vi "Data Channel Page.vi"(8 "error in (no error)":errorcluster, 11 "Node Ptr":T2 format="%.0x") -> (0 "error out":errorcluster)   [LabVIEW 2019, in "DSF System Explorer.lvlib"]
uses:
  DSF System Explorer.lvlib
  <vilib>/NI VeriStand/Custom Device API/Custom Device API.lvlib
  Shared/DSF Shared.lvlib
  DSF Core.lvlibp/Classes/Component User Interface/UI Type.ctl
  <vilib>/NI VeriStand/Custom Device API/Custom Device Item Ref.ctl
panel:
  in  "Tab Control":enum32{"Settings"}(tab)
  in  "Default Value":dbl
  in  "Units":string
  out "Direction":enum16{"Tx", "Rx"}(ring)
  in  "Engine Data Type":T1(ring)
  in  "String Data Type":T1(ring)
  in  "String Offset":u64 format="%d bytes"
  in  "Header":cluster{"Section Name":string}={"Section Name"="Data Channel"}
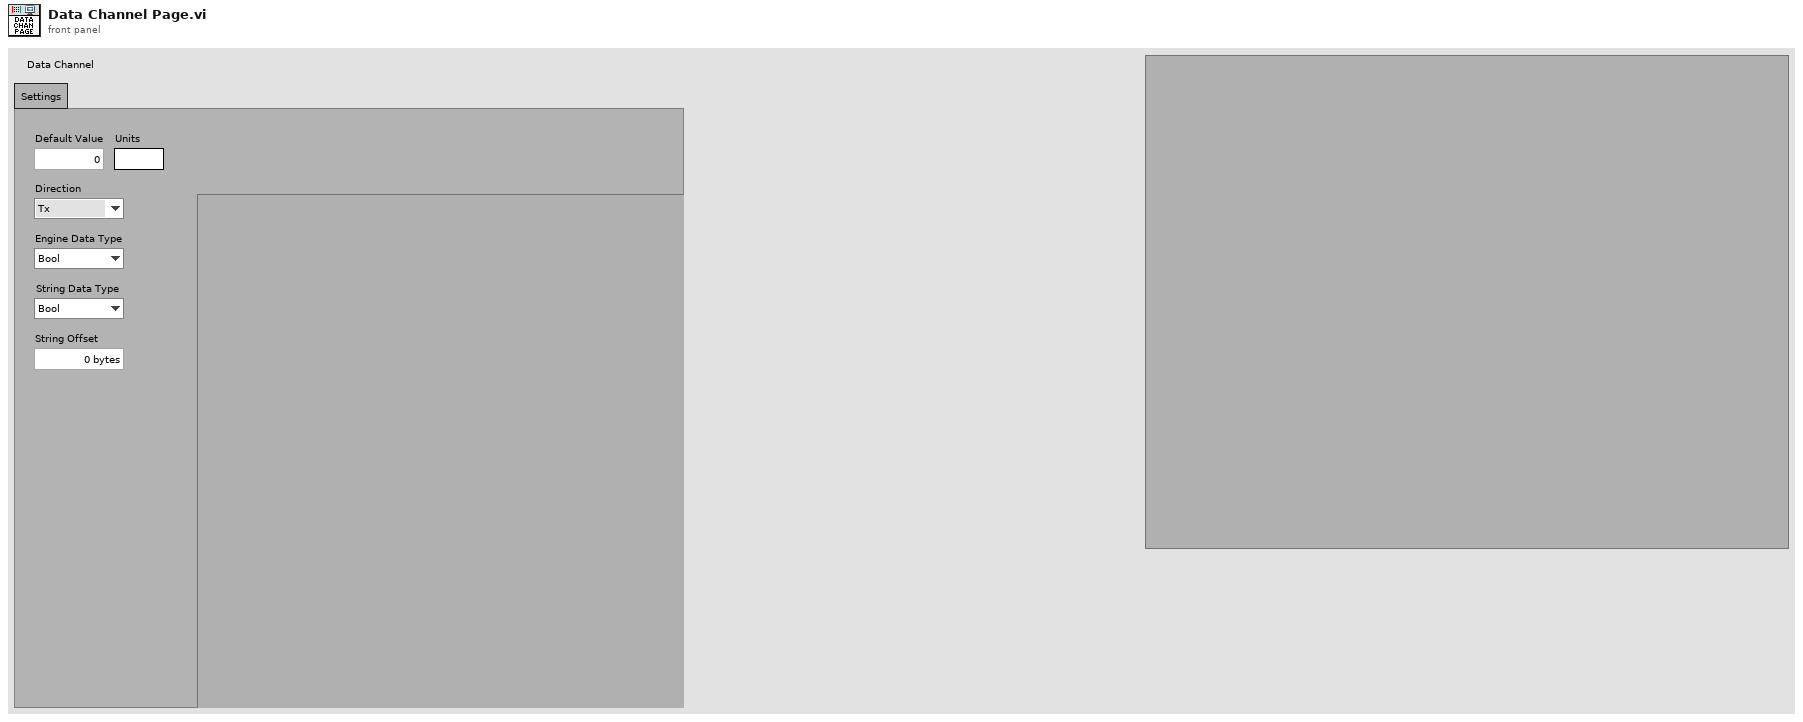
[diagram p1: front panel]
types:
  T1 = enum8{"Bool", "SGL", "DBL", "I8", "I16", "I32", "I64", "U8", "U16", "U32", "U64"}
  T2 = typedef "Custom Device API.lvlib/Custom Device Item Ref.ctl" = u64
  T3 = typedef "DSF Core.lvlibp/Component User Interfaces.lvclass/UI Type.ctl" = enum16{"Plugin", "Thread", "Rx Group", "Tx Group", "Rx Transfer", "Tx Transfer", "Rx Channel", "Tx Channel"}
  T4 = typedef "DSF Core.lvlibp/Channel Configuration.lvclass/Core Channel Configuration.ctl" = cluster{"name":string, "units":string, "engine data type":T5, "string data type":T5, "string offset":u64}
  T5 = typedef "DSF Core.lvlibp/DSF Data Type.ctl" = enum8{"Bool", "SGL", "DBL", "I8", "I16", "I32", "I64", "U8", "U16", "U32", "U64"}
  T6 = typedef "Custom Device API.lvlib/Custom Device Channel.ctl" = cluster{"Type":T7, "Units":string, "Default Value":dbl, "Faultable":bool, "Scalable":bool}
  T7 = typedef "Custom Device API.lvlib/Custom Device Channel Type.ctl" = enum16{"Input", "Output"}
  T8 = typedef "DSF Core.lvlibp/DSF Direction.ctl" = enum8{"Tx", "Rx"}
  T9 = typedef "DSF Core.lvlibp/User Interface Handler.lvclass/User Interface Ref.ctl" = refnum<vi>
  T10 = typedef "DSF Core.lvlibp/DSF Settings Info.ctl" = cluster{"component":string, "values":cluster{"key":string, "value":string}[]}
  T11 = typedef "Custom Device API.lvlib/Custom Device Commands.ctl" = enum16{"Default", "Item renamed", "Shutdown", "Dynamic button pressed"}
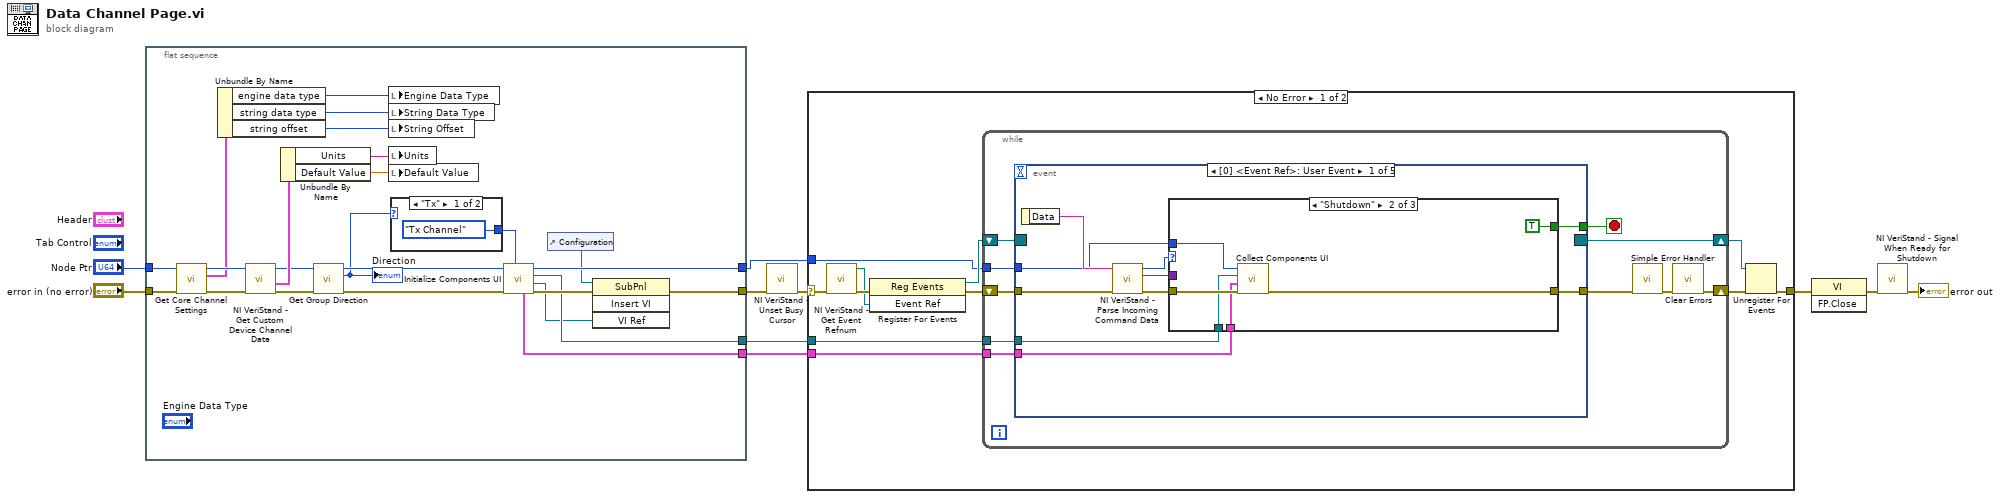
[diagram p0: block diagram]
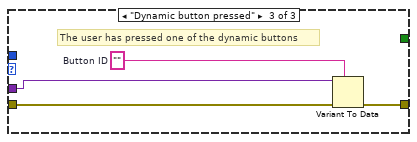
[diagram p3: hidden frame]
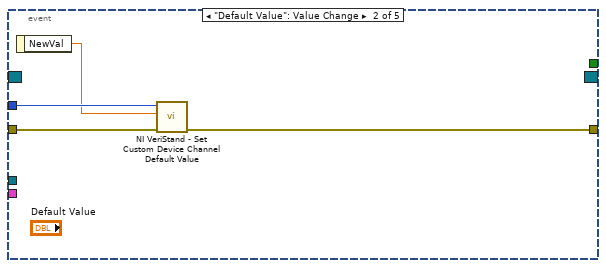
[diagram p4: hidden frame]
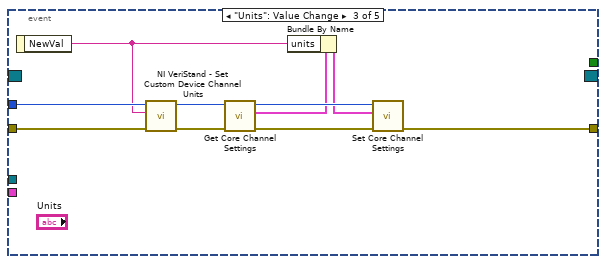
[diagram p5: hidden frame]
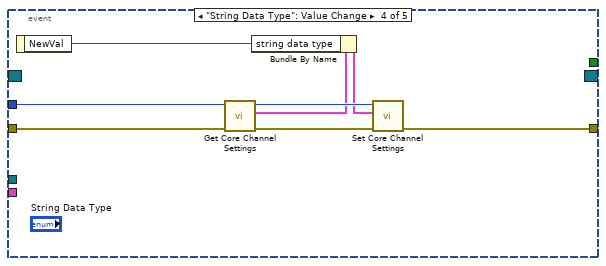
[diagram p6: hidden frame]
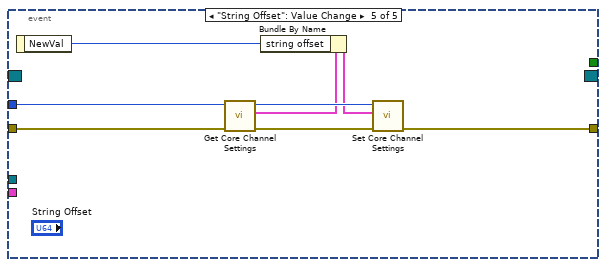
[diagram p7: hidden frame]
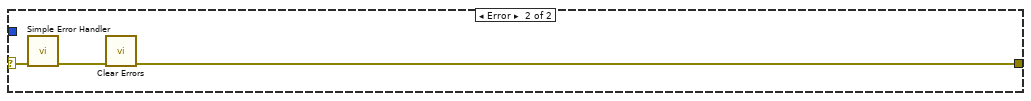
[diagram p8: hidden frame]
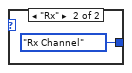
[diagram p9: hidden frame]
diagram:
  n1 = flat-sequence "Initialization code" {
    tunnel: "error in (no error)" -> [w32]
    tunnel: "Node Ptr" -> [w31]
    tunnel: [w19] -> w6
    tunnel: [w14] -> w3
    tunnel: [w15] -> w2
    tunnel: [w11] -> w1
    frame #0 {
      n2 = call "Get Core Channel Settings.vi"("error in (no error)"=w32, "Item Ref in"=w31) -> ("error out"=w30:errorcluster, "channel configuration"=w28:T4, "Item Ref out"=w29:T2)  [unwired: 7 in]
      n3 = Unbundle By Name(w28) -> ("engine data type"=w26:T5, "string data type"=w25:T5, "string offset"=w24:u64)
      n4 = call <vilib>:"NI VeriStand - Get Custom Device Channel Data.vi"("error in (no error)"=w30, "Channel Ref in"=w29) -> ("error out"=w23:errorcluster, "Channel"=w27:T6, "Channel Ref out"=w22:T2)  [unwired: 4 in, 3 out]
      n5 = Unbundle By Name(w27) -> ("Units"=w33:string, "Default Value"=w34:dbl)
      n6 = call "Get Group Direction.vi"("error in (no error)"=w23, "Item Ref in"=w22) -> ("error out"=w18:errorcluster, "direction"=w16:T8, "Item Ref out"=w17:T2)  [unwired: 6 in, 1 out]
      "Direction" <- w16
      n7 = local write "Engine Data Type"(w26) -> ()
      n8 = local write "String Data Type"(w25) -> ()
      n9 = local write "String Offset"(w24) -> ()
      n10 = local write "Units"(w33) -> ()
      n11 = local write "Default Value"(w34) -> ()
      n12 = case shown="\"Tx\"" w16 {
        tunnel: [UI_Type."Tx Channel" ("user interface type") UI_Type."Rx Channel" ("user interface type")] -> w21
        frame "Tx" {
        }
        frame "Rx" {
        }
      }
      n13 = call "Initialize Components UI.vi"("user interface type"=w21, "error in (no error)"=w18, "Item Ref in"=w17) -> ("error out"=w20:errorcluster, "active vi"=w13:T9, "User Interface Handler"=w15:refnum<class "User Interface Handler.lvclass">, "Item Ref out"=w14:T2, "component settings"=w11:T10[])  [unwired: 4 in]
      n14 = control-ref of="Configuration"() -> (w12:refnum<vi>)
      n15 = invoke class="SubPnl" method="Insert VI"(reference=w12, error in=w20, "VI Ref"=w13) -> (error out=w19:errorcluster)  [unwired: 1 in, 3 out]
    }
  }
  n16 = call <vilib>:"NI VeriStand - Unset Busy Cursor.vi"("error in (no error)"=w6) -> ("error out"=w5:errorcluster)  [unwired: 10 out]
  n17 = case shown="No Error" w5 {
    selector: w5 -> [w39 w111]
    tunnel: [w44 w109] -> w10
    tunnel: w3 -> [w40 _]
    tunnel: w2 -> [w38 _]
    tunnel: w1 -> [w37 _]
    frame No Error {
      n18 = call <vilib>:"NI VeriStand - Get Event Refnum.vi"("error in (no error)"=w39) -> ("error out"=w47:errorcluster, "Event Ref"=w43:refnum<user-event>)  [unwired: 9 out]
      n19 = register-events(error in=w47, w43) -> (reference out=w41:refnum<event-registration>, error out=w42:errorcluster)  [unwired: 1 in]
      n20 = while {
        tunnel: w40 -> [w53]
        shift-right: [w50] -> w45
        shift-left: w42 -> [w56]
        shift-right: [w57] -> w46
        shift-left: w41 -> [w55]
        tunnel: w38 -> [w49]
        tunnel: w37 -> [w48]
        stop <- w54 stop-if-true
        n21 = event shown="[0] <Event Ref>: User Event" {
          selector: w55 -> [_ _ _ _ _]
          dyn-events: [_ _ _ _ _] -> w57
          timeout: _ -> [_ _ _ _ _]
          tunnel: w56 -> [w67 w82 w92 w100 w108]
          tunnel: [w63 _ _ _ _] -> w54
          tunnel: [w62 w79 w83 w93 w101] -> w52
          tunnel: w53 -> [w61 w81 w91 w99 w107]
          tunnel: w49 -> [w59 _ _ _ _]
          tunnel: w48 -> [w58 _ _ _ _]
          event User Event {
            n22 = event-data() -> ("Data"=w66:string)  [unwired: 1 out]
            n23 = call <vilib>:"NI VeriStand - Parse Incoming Command Data.vi"("error in (no error)"=w67, "Incoming data"=w66) -> ("error out"=w65:errorcluster, "Outgoing data"=w60:variant, "Action"=w64:T11)  [unwired: 7 out]
            n24 = case shown="\"Shutdown\"" w64 {
              tunnel: w65 -> [w68 w73 w78]
              tunnel: [_ TRUE _] -> w63
              tunnel: [w68 w70 w75] -> w62
              tunnel: w61 -> [_ w72 _]
              tunnel: w60 -> [_ _ w77]
              tunnel: w59 -> [_ w71 _]
              tunnel: w58 -> [_ w69 _]
              frame "Default", Default {
              }
              frame "Shutdown" {
                n25 = call "Collect Components UI.vi"("error in (no error)"=w73, "current component settings"=w69, "User Interface Handler"=w71, "Item Ref in"=w72) -> ("error out"=w70:errorcluster)  [unwired: 6 in, 1 out]
              }
              frame "Dynamic button pressed" {
                w76 = ""  # Button ID
                # "The user has pressed one of the dynamic buttons"
                n26 = Variant To Data(error in=w78, type=w76, Variant=w77) -> (error out=w75:errorcluster)  [unwired: 1 out]
              }
            }
          }
          event "Default Value": Value Change {
            n27 = event-data() -> ("NewVal"=w80:dbl)  [unwired: 1 out]
            n28 = call <vilib>:"NI VeriStand - Set Custom Device Channel Default Value.vi"("error in (no error)"=w82, "Default Value"=w80, "Channel Ref in"=w81) -> ("error out"=w79:errorcluster)  [unwired: 7 in, 1 out]
          }
          event "Units": Value Change {
            n29 = event-data() -> ("NewVal"=w84:string)  [unwired: 1 out]
            n30 = call <vilib>:"NI VeriStand - Set Custom Device Channel Units.vi"("error in (no error)"=w92, "Units"=w84, "Channel Ref in"=w91) -> ("error out"=w90:errorcluster, "Channel Ref out"=w89:T2)  [unwired: 7 in]
            n31 = call "Get Core Channel Settings.vi"("error in (no error)"=w90, "Item Ref in"=w89) -> ("error out"=w88:errorcluster, "channel configuration"=w86:T4, "Item Ref out"=w87:T2)  [unwired: 7 in]
            n32 = Bundle By Name(cluster=w86, "units"=w84) -> (w85:T4)
            n33 = call "Set Core Channel Settings.vi"("error in (no error)"=w88, "channel configuration"=w85, "Item Ref in"=w87) -> ("error out"=w83:errorcluster)  [unwired: 7 in, 1 out]
          }
          event "String Data Type": Value Change {
            n34 = event-data() -> ("NewVal"=w94:T1)  [unwired: 1 out]
            n35 = call "Get Core Channel Settings.vi"("error in (no error)"=w100, "Item Ref in"=w99) -> ("error out"=w98:errorcluster, "channel configuration"=w96:T4, "Item Ref out"=w97:T2)  [unwired: 7 in]
            n36 = Bundle By Name(cluster=w96, "string data type"=w94) -> (w95:T4)
            n37 = call "Set Core Channel Settings.vi"("error in (no error)"=w98, "channel configuration"=w95, "Item Ref in"=w97) -> ("error out"=w93:errorcluster)  [unwired: 7 in, 1 out]
          }
          event "String Offset": Value Change {
            n38 = event-data() -> ("NewVal"=w102:u64)  [unwired: 1 out]
            n39 = call "Get Core Channel Settings.vi"("error in (no error)"=w108, "Item Ref in"=w107) -> ("error out"=w106:errorcluster, "channel configuration"=w104:T4, "Item Ref out"=w105:T2)  [unwired: 7 in]
            n40 = Bundle By Name(cluster=w104, "string offset"=w102) -> (w103:T4)
            n41 = call "Set Core Channel Settings.vi"("error in (no error)"=w106, "channel configuration"=w103, "Item Ref in"=w105) -> ("error out"=w101:errorcluster)  [unwired: 7 in, 1 out]
          }
        }
        n42 = call <vilib>:"Simple Error Handler.vi"("error in (no error)"=w52) -> ("error out"=w51:errorcluster)  [unwired: 1 in, 7 out]
        n43 = call <vilib>:"Clear Errors.vi"("error in (no error)"=w51) -> ("error out"=w50:errorcluster)  [unwired: 1 in, 5 out]
      }
      n44 = Unregister For Events(event registration refnum=w46, error in=w45) -> (error out=w44:errorcluster)
    }
    frame Error {
      n45 = call <vilib>:"Simple Error Handler.vi"("error in (no error)"=w111) -> ("error out"=w110:errorcluster)  [unwired: 1 in, 7 out]
      n46 = call <vilib>:"Clear Errors.vi"("error in (no error)"=w110) -> ("error out"=w109:errorcluster)  [unwired: 1 in, 5 out]
    }
  }
  n47 = invoke class="VI" method="FP.Close"(error in=w10) -> (error out=w9:errorcluster)  [unwired: 2 in, 2 out]
  n48 = call <vilib>:"NI VeriStand - Signal When Ready for Shutdown.vi"("error in (no error)"=w9) -> ("error out"=→"error out":errorcluster)  [unwired: 10 out]
